vi "New Back Legs.vi"(8 "isDualActing":bool, 10 "Engage Leg 1/2":bool, 11 "New state":string) -> (1 "Old state":string, 2 "Claw":T1)   [LabVIEW 2012]
uses:
  <vilib>/Rock Robotics/WPI/Solenoid/WPI_SolenoidValue.ctl
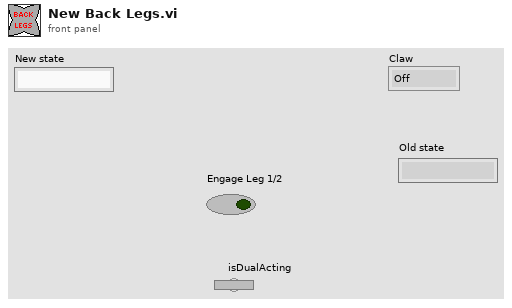
[diagram p1: front panel]
types:
  T1 = typedef "WPI_SolenoidValue.ctl" = enum16{"Off", "On", "Forward", "Reverse"}
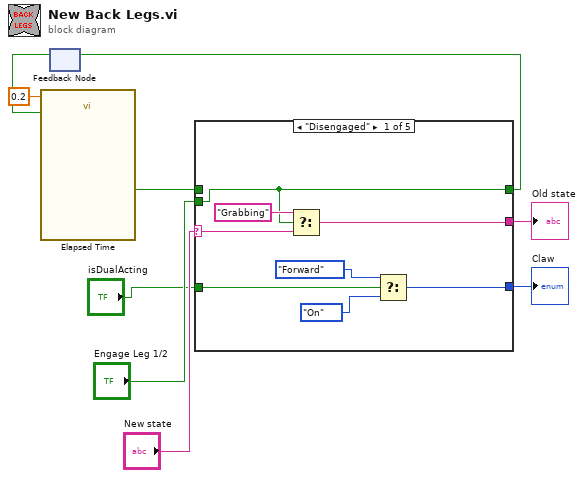
[diagram p0: block diagram]
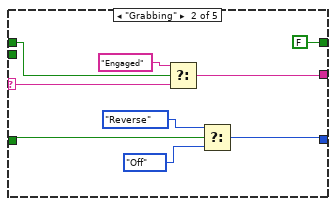
[diagram p2: hidden frame]
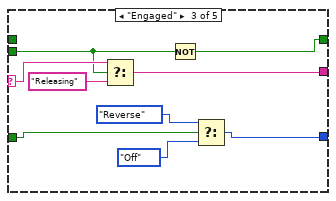
[diagram p3: hidden frame]
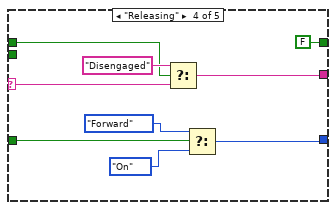
[diagram p4: hidden frame]
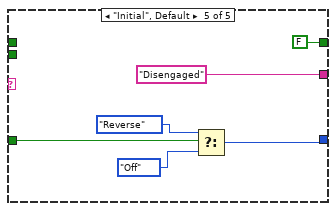
[diagram p5: hidden frame]
diagram:
  n1 = feedback #1() -> (w2:bool)  [unwired: 1 in]
  n2 = call "Elapsed Time"("Time Target (s)"=0.2, "Reset"=w2) -> ("Time has Elapsed"=w4:bool)  [unwired: 10 in, 7 out]
  n3 = case shown="\"Disengaged\"" "New state" {
    selector: "New state" -> [w15 w25 w33 w44 _]
    tunnel: [w17 w26 w35 w43 "Disengaged"] -> w7
    tunnel: "Engage Leg 1/2" -> [w14 _ w31 _ _]
    tunnel: [w10 w19 w27 w37 w45] -> w8
    tunnel: w4 -> [_ w23 _ w41 _]
    tunnel: [w14 FALSE ("Time has Elapsed") w32 FALSE ("Time has Elapsed") FALSE ("Time has Elapsed")] -> w3
    tunnel: "isDualActing" -> [w13 w18 w28 w36 w46]
    frame "Disengaged" {
      n4 = Select(t="Grabbing", s=w14, f=w15) -> (s? t:f=w17:string)
      n5 = Select(t=WPI_SolenoidValue."Forward" ("Foot"), s=w13, f=WPI_SolenoidValue."On" ("Foot")) -> (s? t:f=w10:T1)
    }
    frame "Grabbing" {
      n6 = Select(t="Engaged", s=w23, f=w25) -> (s? t:f=w26:string)
      n7 = Select(t=WPI_SolenoidValue."Reverse" ("Foot"), s=w18, f=WPI_SolenoidValue."Off" ("Foot")) -> (s? t:f=w19:T1)
    }
    frame "Engaged" {
      n8 = Select(t=w33, s=w31, f="Releasing") -> (s? t:f=w35:string)
      n9 = Not(x=w31) -> (.not. x?=w32:bool)
      n10 = Select(t=WPI_SolenoidValue."Reverse" ("Foot"), s=w28, f=WPI_SolenoidValue."Off" ("Foot")) -> (s? t:f=w27:T1)
    }
    frame "Releasing" {
      n11 = Select(t="Disengaged", s=w41, f=w44) -> (s? t:f=w43:string)
      n12 = Select(t=WPI_SolenoidValue."Forward" ("Foot"), s=w36, f=WPI_SolenoidValue."On" ("Foot")) -> (s? t:f=w37:T1)
    }
    frame "Initial", Default {
      n13 = Select(t=WPI_SolenoidValue."Reverse" ("Foot"), s=w46, f=WPI_SolenoidValue."Off" ("Foot")) -> (s? t:f=w45:T1)
    }
  }
  "Claw" <- w8
  "Old state" <- w7
  n14 = feedback-in #1(w3) -> ()
